vi "iow_Get Current Pin Status.vi"() -> ()   [LabVIEW 2011]
panel:
  out "?":u8 format="%02x"
  out "?":u8 format="%02x"
  out "arrayout":u8[](array[numeric]) format="%.0x"
  out "Error Connect":errorcluster caption="error"
  out "?":u8 format="%02x"
  out "Flags":u8 format="%02x"
  out "ReportID":u8 format="%02x"
  out "Error Read":errorcluster caption="error"
  out "Error Write":errorcluster caption="error"
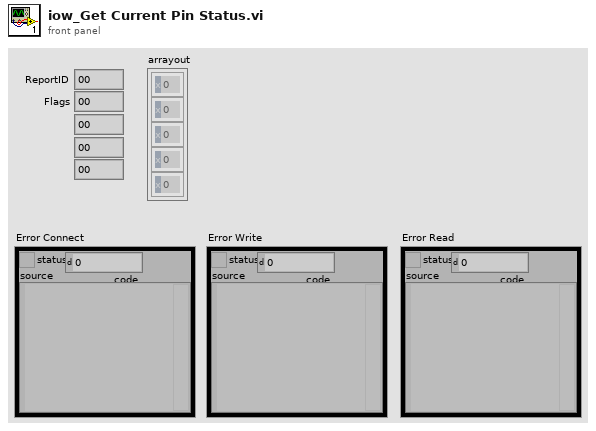
[diagram p1: front panel]
types:
  T1 = typedef "IOWarrior_Handle.ctl" = cluster{"Handle":u32, "Serial Number":string, "type of Warrior":T2, "Root Handle":bool, "Revision":u16}
  T2 = typedef "IOWarrior_Type.ctl" = enum16{"invalid", "IOW24", "IOW40", "IOW56", "IOPV1", "IOPV2"}
  T3 = cluster{"arrayout[0]":u8, "arrayout[1]":u8, "arrayout[2]":u8, "arrayout[3]":u8, "arrayout[4]":u8}
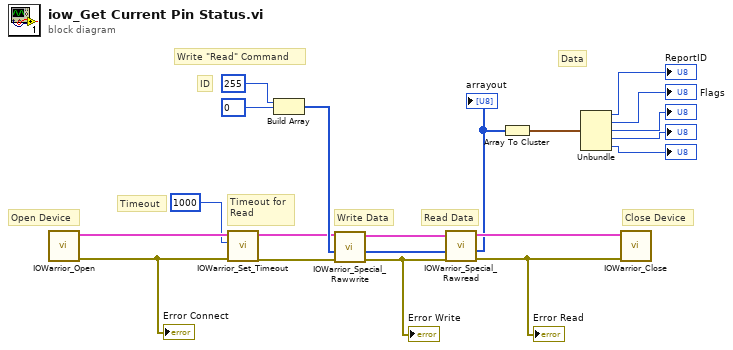
[diagram p0: block diagram]
diagram:
  # "Data"
  # "Timeout"
  # "Open Device"
  # "Close Device"
  # "Write Data"
  # "Read Data"
  # "ID"
  # "Write \"Read\" Command"
  # "Timeout for\nRead"
  n1 = call "IOWarrior_Open.vi"() -> ("err out"=w14:errorcluster, "IOWarriorHandle"=w20:T1)  [unwired: 9 in, 1 out]
  "Error Connect" <- w14
  n2 = call "IOWarrior_Set_Timeout.vi"("err in"=w14, "timeout_ms(1000)"=1000, "devHandle"=w20) -> ("err out"=w2:errorcluster, "devHandleout"=w3:T1)  [unwired: 6 in, 1 out]
  n3 = Build Array(u8 255, u8 0) -> (w11:u8[])
  n4 = call "IOWarrior_Special_Rawwrite.vi"("err in"=w2, "Array_in"=w11, "devHandle"=w3) -> ("err out"=w4:errorcluster, "array_out"=w10:u8[], "devHandleout"=w12:T1)  [unwired: 6 in]
  "Error Write" <- w4
  n5 = call "IOWarrior_Special_Rawread.vi"("err in"=w4, "array"=w10, "devHandle"=w12) -> ("err out"=w16:errorcluster, "arrayout"=w13:u8[], "devHandleout"=w18:T1)  [unwired: 6 in]
  "Error Read" <- w16
  "arrayout" <- w13
  n6 = Array To Cluster(array=w13) -> (cluster=w15:T3)
  n7 = Unbundle(w15) -> ("arrayout[0]"=→"ReportID":u8, "arrayout[1]"=→"Flags":u8, "arrayout[2]"=→"?":u8, "arrayout[3]"=→"?":u8, "arrayout[4]"=→"?":u8)
  n8 = call "IOWarrior_Close.vi"("err in"=w16, "devHandle"=w18) -> ()  [unwired: 8 in, 2 out]
